vi "Initialise Transient Mode.vi"(8 "error in":errorcluster, 9 "Data Size":T1, 10 "Maximum Waveform Length":i32=10000, 11 "configuration file path":path) -> (0 "error out":errorcluster)   [LabVIEW 2017, in "DTACQ - Network Enabled Device Driver.lvlib"]
doc: "Prepares the Dtacq device for transient capture mode"
uses:
  DTACQ - Network Enabled Device Driver.lvlib
  Communications/Typedefs/Data Size--Enum.ctl
  Driver Global Settings--Typedef.ctl
  Communications/Typedefs/DTACQ Connection Data--Cluster.ctl
  FGV Operaions--Enum.ctl
  Communications/Communications Library.lvlib
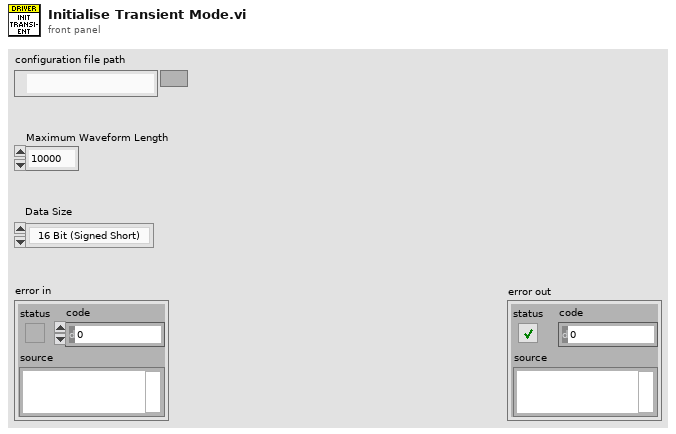
[diagram p1: front panel]
types:
  T1 = typedef "Communications Library.lvlib/Data Size--Enum.ctl" = enum16{"16 Bit (Signed Short)", "32 Bit (Signed Long)"}
  T2 = typedef "DTACQ - Network Enabled Device Driver.lvlib/FGV Operaions--Enum.ctl" = enum16{"Get Driver Settings", "Set Driver Settings", "Search Variable Names", "Close Connections", "Open Connections", "Get Variable References", "Set Variable References", "Clear"}
  T3 = typedef "DTACQ - Network Enabled Device Driver.lvlib/Driver Global Settings--Typedef.ctl" = cluster{"Waveform Length":i32, "Data Size":T1, "DTACQ Connection Data":T4}
  T4 = typedef "Communications Library.lvlib/DTACQ Connection Data--Cluster.ctl" = cluster{"Description":string, "Address":string, "Port":u16, "timeout (ms)":i32, "Termination Character":string, "TCP Connection Reference":refnum<k5>, "Open Connection":bool}
  T5 = typedef "Communications Library.lvlib/DTACQ Module Carrier Configuration--Cluster.ctl" = cluster{"Name":string, "IP":string, "Control Port":i32, "Timeout (ms)":i32, "Continuous Capture Port (Multiplexed)":i32, "Start HIL Shot Port":i32, "AWG Upload Port (Multiplexed)":i32, "Download Captured Data Port (Multiplexed)":i32, "Module Slots":i32, "Module Configurations":T6[]}
  T6 = typedef "Communications Library.lvlib/DTACQ Module Configuration--Cluster.ctl" = cluster{"Name":string, "Position":string, "Module Type":T7, "Control Port":i32, "Timeout (ms)":i32, "Channels":i32}
  T7 = typedef "Communications Library.lvlib/DTACQ Device Type--Enum.ctl" = enum16{"Carrier", "Analog In Module", "Analog Out Module", "Generic Module"}
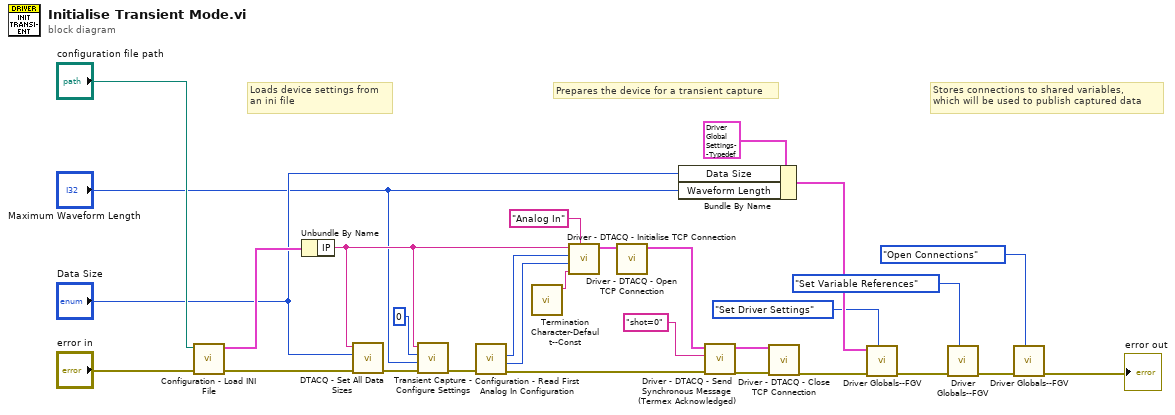
[diagram p0: block diagram]
diagram:
  # "Stores connections to shared variables,\nwhich will be used to publish captured data"
  # "Prepares the device for a transient capture"
  # "Loads device settings from\nan ini file"
  n1 = call "Configuration - Load INI File.vi"("error in"="error in", "configuration file path"="configuration file path") -> ("error out"=w26:errorcluster, "Carrier Configuration Out"=w27:T5)  [unwired: 8 in]
  n2 = Unbundle By Name(w27) -> ("IP"=w3:string)
  n3 = call "DTACQ - Set All Data Sizes.vi"("error in"=w26, "Analog In Data Size"="Data Size", "Address"=w3) -> ("error out"=w5:errorcluster)  [unwired: 7 in, 1 out]
  n4 = call "Transient Capture - Configure Settings.vi"("error in"=w5, "Samples to Read (Post Trigger)"="Maximum Waveform Length", "Samples to Read (Pre Trigger)"=0, "Address"=w3) -> ("error out"=w4:errorcluster)  [unwired: 7 in]
  n5 = call "Configuration - Read First Analog In Configuration.vi"("error in"=w4) -> ("error out"=w19:errorcluster, "Timeout (ms)"=w22:i32, "Analog In Control Port"=w23:i32)  [unwired: 6 in, 2 out]
  n6 = call "Termination Character-Default--Const.vi"() -> ("Termination Character"=w21:string)  [unwired: 11 in]
  n7 = call "Driver - DTACQ - Initialise TCP Connection.vi"("Description"="Analog In", "Termination Character"=w21, "timeout (ms)"=w22, "Port"=w23, "Address"=w3) -> ("DTACQ Connection Data Out"=w24:T4)  [unwired: 6 in]
  n8 = call "Driver - DTACQ - Open TCP Connection.vi"("DTACQ Connection Data In"=w24) -> ("DTACQ Connection Data Out"=w20:T4)  [unwired: 9 in, 1 out]
  n9 = Bundle By Name(cluster=T3 {"Waveform Length"=0, "Data Size"=enum."16 Bit (Signed Short)", "DTACQ Connection Data"={"Description"="", "Address"="", "Port"=0, "timeout (ms)"=5000, "Termination Character"="\n", "TCP Connection Reference"=refnum, "Open Connection"=FALSE}} ("Driver Settings In"), "Data Size"="Data Size", "Waveform Length"="Maximum Waveform Length") -> (w15:T3)
  n10 = call "Driver - DTACQ - Send Synchronous Message (Termex Acknowledged).vi"("error in"=w19, "Message to Send"="shot=0", "DTACQ Connection Data In"=w20) -> ("error out"=w16:errorcluster, "DTACQ Connection Data Out"=w17:T4)  [unwired: 5 in, 2 out]
  n11 = call "Driver - DTACQ - Close TCP Connection.vi"("error in"=w16, "DTACQ Connection Data In"=w17) -> ("error out"=w10:errorcluster)  [unwired: 8 in, 1 out]
  n12 = call "Driver Globals--FGV.vi"(7:FGV_Operaions--Enum."Set Driver Settings", "error in"=w10, "Driver Settings In"=w15) -> ("error out"=w9:errorcluster)  [unwired: 5 in, 3 out]
  n13 = call "Driver Globals--FGV.vi"(7:FGV_Operaions--Enum."Set Variable References", "error in"=w9) -> ("error out"=w8:errorcluster)  [unwired: 6 in, 3 out]
  n14 = call "Driver Globals--FGV.vi"(7:FGV_Operaions--Enum."Open Connections", "error in"=w8) -> ("error out"=→"error out":errorcluster)  [unwired: 6 in, 3 out]
